vi "STM_Status - Copy.vi"() -> ()   [LabVIEW 2014]
uses:
  <userlib>/Nanonis Prog Interface V5/Nanonis Prog Interface.lvlib
panel:
  in  "Emission Current":u16(ring) items=["10", "1", "0.1"]
  out "STM [mBar]":dbl=2.950733268836103e-10 format="%#.2g"
  out "Prep [mBar]":dbl=6.164446730849704e-10 format="%#.2g"
  out "Pressure":cluster{timestamp[], dbl[]}[](graph)
  in  "Resolution P":dbl=0.1
  in  "force update":dbl=20.0
  out "Cryo [K]":dbl=4.220996172878398 format="%#.2g"
  out "STM [K]":dbl=4.621647438892101 format="%#.2g"
  in  "Resolution Temp":dbl=0.01
  out "Temperature":cluster{timestamp[], dbl[]}[](graph)=[{[timestamp(3556847215.1879015 s since 1904-01-01), timestamp(3556847235.26605 s since 1904-01-01), timestamp(3556847255.298196 s since 1904-01-01), timestamp(3556847275.3973455 s since 1904-01-01), timestamp(3556847295.4834943 s since 1904-01-01), timestamp(3556847315.6116457 s since 1904-01-01), timestamp(3556847335.637791 s since 1904-01-01), timestamp(3556847355.736941 s since 1904-01-01), timestamp(3556847375.8420906 s since 1904-01-01), timestamp(3556847395.9452405 s since 1904-01-01), timestamp(3556847416.073392 s since 1904-01-01), timestamp(3556847436.1085377 s since 1904-01-01), timestamp(3556847456.3296943 s since 1904-01-01)], [4.2207562780232655, 4.2205274552383685, 4.2209592659776085, 4.220173148990788, 4.220638175940738, 4.221992659199721, 4.220866998725635, 4.220940812527213, 4.220892833556188, 4.220593887659791, 4.220715680432397, 4.220782112853818, 4.220999863568477]}, {[timestamp(3556847215.1879015 s since 1904-01-01), timestamp(3556847235.26605 s since 1904-01-01), timestamp(3556847255.298196 s since 1904-01-01), timestamp(3556847275.3973455 s since 1904-01-01), timestamp(3556847295.4834943 s since 1904-01-01), timestamp(3556847315.6116457 s since 1904-01-01), timestamp(3556847335.637791 s since 1904-01-01), timestamp(3556847355.736941 s since 1904-01-01), timestamp(3556847375.8420906 s since 1904-01-01), timestamp(3556847395.9452405 s since 1904-01-01), timestamp(3556847416.073392 s since 1904-01-01), timestamp(3556847436.1085377 s since 1904-01-01), timestamp(3556847456.3296943 s since 1904-01-01)], [4.621765262027122, 4.621248919464823, 4.621089511693913, 4.621113769398182, 4.621619715801508, 4.623789047640425, 4.622160316068075, 4.621664765823721, 4.621682092755342, 4.621900412093764, 4.621796450504039, 4.62191427363906, 4.621799915890364]}]
  in  "Clear chart":bool
  in  "stop":bool
  in  "refresh":dbl=0.3
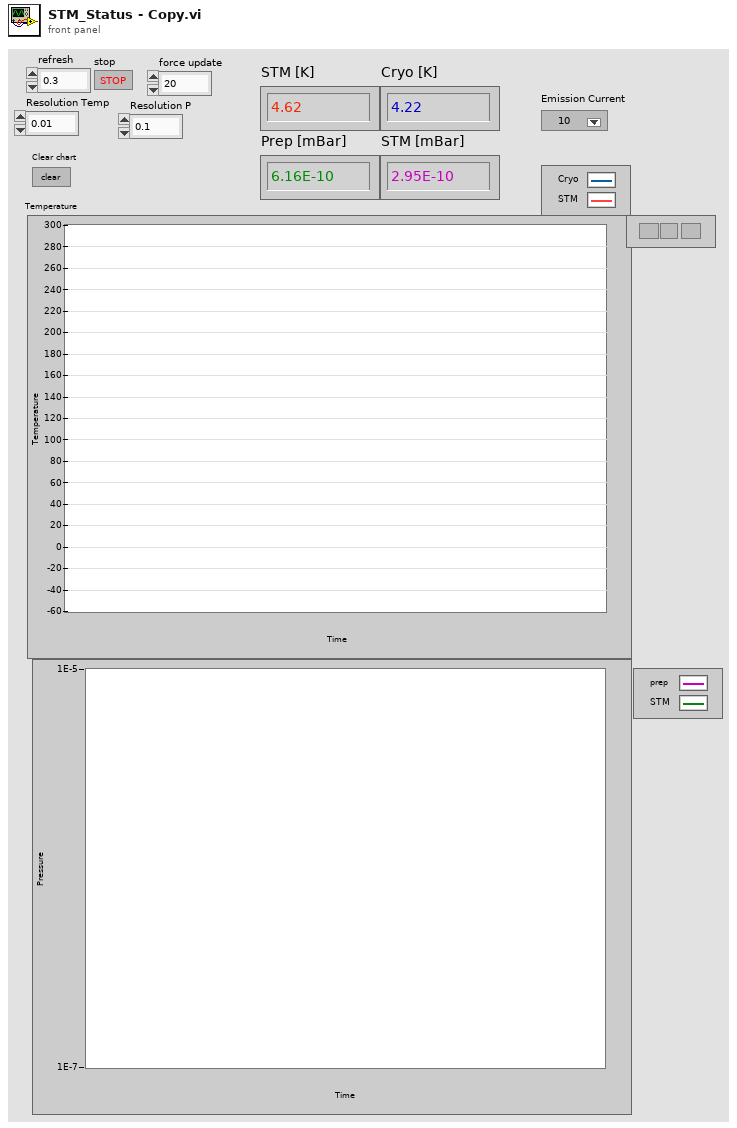
[diagram p1: front panel]
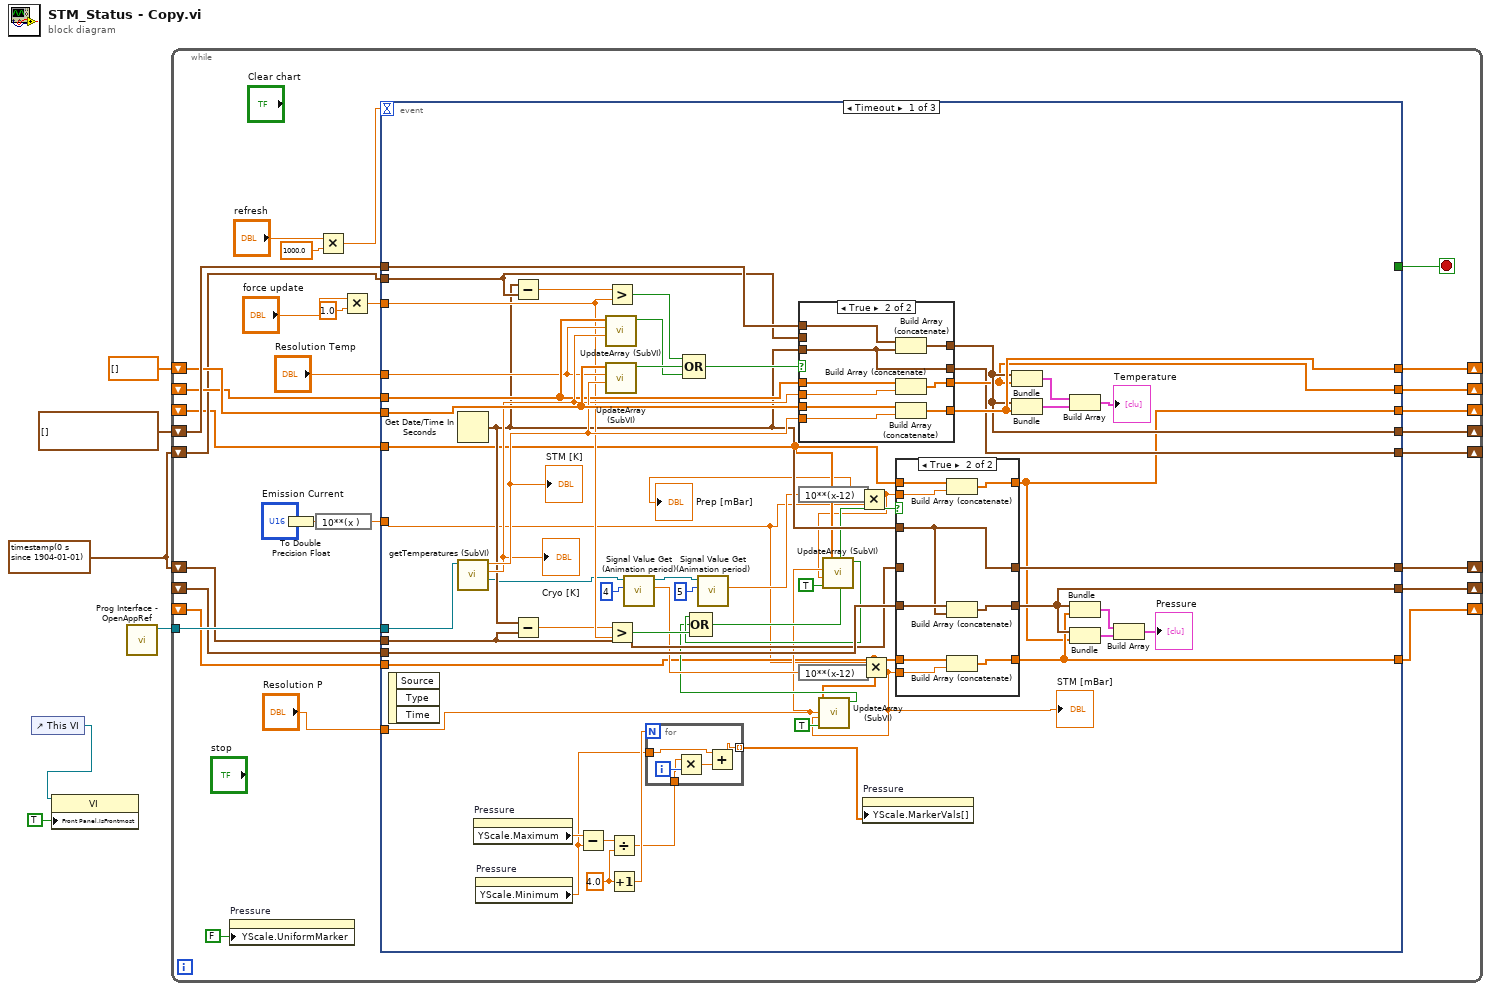
[diagram p0: block diagram]
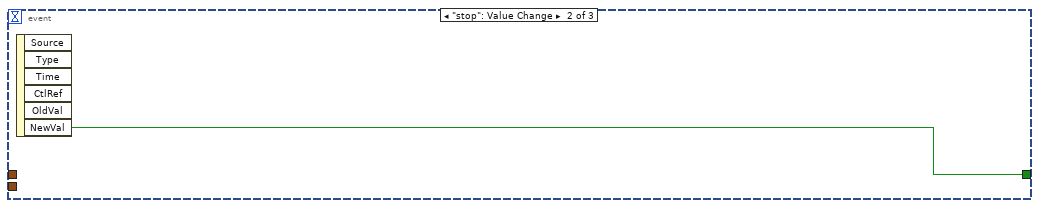
[diagram p4: hidden frame]
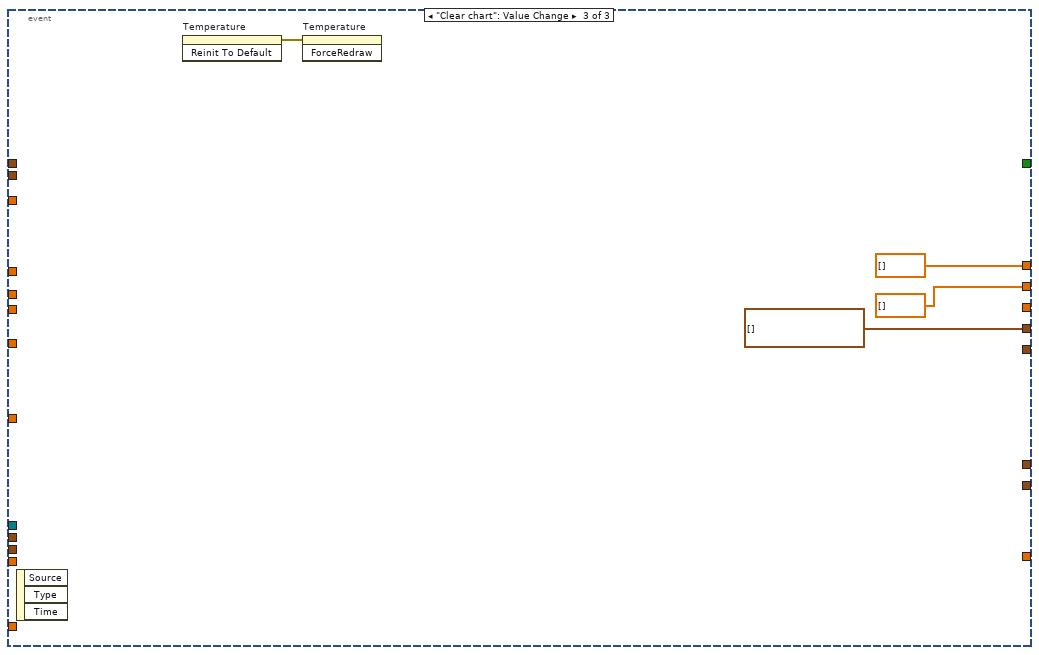
[diagram p5: hidden frame]
diagram:
  w3 = timestamp(0 s since 1904-01-01) ("seconds since 1Jan1904")
  n1 = control-ref of="This VI"() -> (w2:refnum<vi>)
  n2 = property class="VI"(reference=w2, "Front Panel.IsFrontmost"=TRUE ("Front Panel Window:Is Frontmost")) -> ()  [unwired: 1 in, 2 out]
  n3 = call <userlib>:"Prog Interface - OpenAppRef.vi"() -> ("Application reference"=w4:refnum<vi>)  [unwired: 6 in, 1 out]
  n4 = while {
    tunnel: w4 -> [w26]
    shift-right: [w34] -> _
    shift-left: timestamp[] [] -> [w29]
    shift-right: [w33] -> _
    shift-left: dbl[] [] -> [w28]
    shift-right: [w32] -> _
    shift-left: _ -> [w27]
    shift-right: [w24] -> _
    shift-left: w3 -> [w23]
    shift-right: [w19] -> _
    shift-left: _ -> [w18]
    shift-right: [w17] -> _
    shift-left: w3 -> [w16]
    shift-right: [w15] -> _
    shift-left: _ -> [w14]
    shift-right: [w13] -> _
    shift-left: _ -> [w12]
    stop <- w31 stop-if-true
    n5 = property on="Pressure" class="XYGraph (strict)"("YScale.UniformMarker"=FALSE ("Y Scale.Uniform Marker Spacing?")) -> ()  [unwired: 2 in, 2 out]
    n6 = To Double Precision Float(number="Emission Current") -> (double precision float=w7:dbl)
    n7 = expression code="10**(x )"(w7) -> (w8:dbl)
    n8 = Multiply(x="refresh", y=1000.0) -> (x*y=w30:dbl)
    n9 = Multiply(x="force update", y=1.0) -> (x*y=w20:dbl)
    n10 = event shown="[0] Timeout" {
      selector: _ -> [_ _ _]
      dyn-events: _ -> [_ _ _]
      timeout: w30 -> [_ _ _]
      tunnel: [w89 _ timestamp[] []] -> w34
      tunnel: [w90 _ dbl[] []] -> w33
      tunnel: [w88 _ dbl[] []] -> w32
      tunnel: [_ w127 _] -> w31
      tunnel: w29 -> [w92 _ _]
      tunnel: w28 -> [w87 _ _]
      tunnel: w27 -> [w84 _ _]
      tunnel: w26 -> [w91 _ _]
      tunnel: "Resolution Temp" -> [w83 _ _]
      tunnel: [w78 _ _] -> w24
      tunnel: w23 -> [w76 _ _]
      tunnel: w20 -> [w70 _ _]
      tunnel: [w62 _ _] -> w19
      tunnel: w18 -> [w72 _ _]
      tunnel: [w68 _ _] -> w17
      tunnel: w16 -> [w67 _ _]
      tunnel: [w48 _ _] -> w15
      tunnel: w14 -> [w53 _ _]
      tunnel: [w47 _ _] -> w13
      tunnel: w12 -> [w54 _ _]
      tunnel: "Resolution P" -> [w55 _ _]
      tunnel: w8 -> [w44 _ _]
      event Timeout {
        w41 = 4.0 ("y")
        n11 = event-data() -> ()  [unwired: 1 in, 3 out]
        n12 = Get Date/Time In Seconds() -> (seconds since 1Jan1904=w69:timestamp)
        n13 = call "getTemperatures (SubVI).vi"("Application in"=w91) -> ("Application ref out"=w59:refnum<vi>, "TCryo"=w85:dbl, "TSTM"=w86:dbl)  [unwired: 7 in, 1 out]
        "STM [K]" <- w86
        "Cryo [K]" <- w85
        n14 = property on="Pressure" class="XYGraph (strict)"() -> ("YScale.Maximum"=w43:dbl)  [unwired: 2 in, 2 out]
        n15 = property on="Pressure" class="XYGraph (strict)"() -> ("YScale.Minimum"=w39:dbl)  [unwired: 2 in, 2 out]
        n16 = Subtract(x=w69, y=w76) -> (x-y=w79:dbl)
        n17 = Subtract(x=w69, y=w67) -> (x-y=w66:dbl)
        n18 = Subtract(x=w43, y=w39) -> (x-y=w42:dbl)
        n19 = call "UpdateArray (SubVI).vi"("Temp1"=w85, "Resolution"=w83, "Array"=w84) -> ("x > y?"=w80:bool)  [unwired: 8 in]
        n20 = call "UpdateArray (SubVI).vi"("Temp1"=w86, "Resolution"=w83, "Array"=w87) -> ("x > y?"=w81:bool)  [unwired: 8 in]
        n21 = Greater?(x=w79, y=w70) -> (0:w77:bool)
        n22 = Greater?(x=w66, y=w70) -> (0:w71:bool)
        n23 = Divide(x=w42, y=w41) -> (x/y=w38:dbl)
        n24 = Increment(x=w41) -> (x+1=w40:dbl)
        n25 = call <userlib>:"Signal Value Get (Animation period).vi"("Signal index (0-47)"=i8 4, "Application ref in"=w59) -> ("Signal value"=w60:sgl, "Application ref out"=w75:refnum<vi>)  [unwired: 6 in, 1 out]
        n26 = for {
          N: w40 -> [_]
          tunnel: w39 -> [w100]
          tunnel: w38 -> [w98]
          tunnel: [w96] -> w37 mode=indexing
          i -> [w99]
          n27 = Multiply(x=w98, y=w99) -> (x*y=w97:dbl)
          n28 = Add(x=w100, y=w97) -> (x+y=w96:dbl)
        }
        n29 = Compound Arithmetic op=OR(w77, w81, w80) -> (w82:bool)
        n30 = call <userlib>:"Signal Value Get (Animation period).vi"("Signal index (0-47)"=i8 5, "Application ref in"=w75) -> ("Signal value"=w58:sgl)  [unwired: 6 in, 2 out]
        n31 = case shown="True" w82 {
          tunnel: w69 -> [_ w118]
          tunnel: w92 -> [w117 w126]
          tunnel: [w115 w125] -> w90
          tunnel: [w117 w124] -> w89
          tunnel: [w116 w123] -> w88
          tunnel: w87 -> [w115 w122]
          tunnel: w86 -> [_ w121]
          tunnel: w85 -> [_ w120]
          tunnel: w84 -> [w116 w119]
          tunnel: [w114 w118] -> w78
          tunnel: w76 -> [w114 _]
          frame False {
          }
          frame True {
            n32 = Build Array (concatenate)(w126, w118) -> (w124:timestamp[])
            n33 = Build Array (concatenate)(w119, w120) -> (w123:dbl[])
            n34 = Build Array (concatenate)(w122, w121) -> (w125:dbl[])
          }
        }
        n35 = expression code="10**(x-12)"(w58) -> (w52:sgl)
        n36 = expression code="10**(x-12)"(w60) -> (w51:sgl)
        n37 = Multiply(x=w52, y=w44) -> (x*y=w46:dbl)
        "Prep [mBar]" <- w46
        n38 = call "UpdateArray (SubVI).vi"("log"=TRUE, "Temp1"=w46, "Resolution"=w55, "Array"=w54) -> ("x > y?"=w57:bool)  [unwired: 7 in]
        n39 = Multiply(x=w44, y=w51) -> (x*y=w45:dbl)
        "STM [mBar]" <- w45
        n40 = call "UpdateArray (SubVI).vi"("log"=TRUE, "Temp1"=w45, "Resolution"=w55, "Array"=w53) -> ("x > y?"=w56:bool)  [unwired: 7 in]
        n41 = Compound Arithmetic op=OR(w57, w56, w71) -> (w61:bool)
        n42 = property on="Pressure" class="XYGraph (strict)"("YScale.MarkerVals[]"=w37) -> ()  [unwired: 2 in, 2 out]
        n43 = case shown="True" w61 {
          tunnel: w69 -> [_ w106]
          tunnel: w72 -> [w104 w113]
          tunnel: [w102 w112] -> w47
          tunnel: [w104 w111] -> w62
          tunnel: [w103 w110] -> w48
          tunnel: w54 -> [w102 w109]
          tunnel: w46 -> [_ w105]
          tunnel: w45 -> [_ w108]
          tunnel: w53 -> [w103 w107]
          tunnel: [w101 w106] -> w68
          tunnel: w67 -> [w101 _]
          frame False {
          }
          frame True {
            n44 = Build Array (concatenate)(w109, w105) -> (w112:dbl[])
            n45 = Build Array (concatenate)(w113, w106) -> (w111:timestamp[])
            n46 = Build Array (concatenate)(w107, w108) -> (w110:dbl[])
          }
        }
        n47 = Bundle(w89, w88) -> (w95:cluster{timestamp[], dbl[]})  [unwired: 1 in]
        n48 = Bundle(w89, w90) -> (w94:cluster{timestamp[], dbl[]})  [unwired: 1 in]
        n49 = Build Array(w95, w94) -> (→"Temperature":cluster{timestamp[], dbl[]}[])
        n50 = Bundle(w62, w48) -> (w65:cluster{timestamp[], dbl[]})  [unwired: 1 in]
        n51 = Bundle(w62, w47) -> (w64:cluster{timestamp[], dbl[]})  [unwired: 1 in]
        n52 = Build Array(w65, w64) -> (→"Pressure":cluster{timestamp[], dbl[]}[])
      }
      event "stop": Value Change {
        n53 = event-data() -> ("NewVal"=w127:bool)  [unwired: 1 in, 5 out]
      }
      event "Clear chart": Value Change {
        n54 = event-data() -> ()  [unwired: 1 in, 3 out]
        n55 = invoke on="Temperature" class="XYGraph (strict)" method="Reinit To Default"() -> (error out=w128:errorcluster)  [unwired: 3 in, 2 out]
        n56 = invoke on="Temperature" class="XYGraph (strict)" method="ForceRedraw"(error in=w128) -> ()  [unwired: 2 in, 3 out]
      }
    }
  }
